vi "Board Info Report_v2.vi"(8 "error in (no error)":errorcluster, 11 "ControlBoard VISA":refnum<visa-resource-name>="ControlBoard") -> (0 "error out":errorcluster, 3 "Report":string)   [LabVIEW 2022 SP3]
uses:
  SupportVIs/VISA Flush IO Buffer Mask.ctl
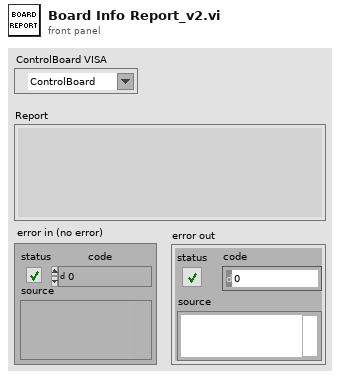
[diagram p1: front panel]
types:
  T1 = typedef "VISA Flush IO Buffer Mask.ctl" = u16
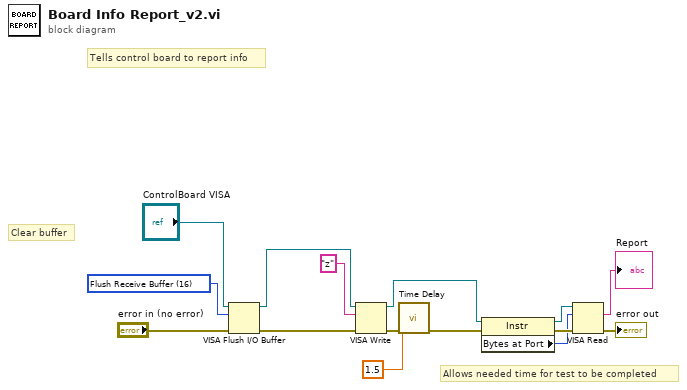
[diagram p0: block diagram]
diagram:
  w14 = T1 16 items=["Flush Receive Buffer"=16, "Write Transmit Buffer to Device"=32, "Flush Receive Buffer (No I/O)"=64, "Flush Transmit Buffer"=128] ("Mask")
  # "Allows needed time for test to be completed"
  # "Tells control board to report info"
  # "Clear buffer"
  n1 = VISA Flush I/O Buffer(VISA resource name="ControlBoard VISA", mask (16)=w14, error in (no error)="error in (no error)") -> (VISA resource name out=w12:refnum<visa-resource-name>, error out=w9:errorcluster)
  n2 = VISA Write(VISA resource name=w12, write buffer="z", error in (no error)=w9) -> (VISA resource name out=w7:refnum<visa-resource-name>, error out=w13:errorcluster)  [unwired: 1 out]
  n3 = call "Time Delay"("error in (no error)"=w13, "Delay Time (s)"=1.5) -> ("error out"=w8:errorcluster)  [unwired: 9 in]
  n4 = property class="Instr"(reference=w7, error in=w8) -> (reference out=w6:refnum<visa-resource-name>, error out=w5:errorcluster, "Bytes at Port"=w4:u32)
  n5 = VISA Read(VISA resource name=w6, byte count=w4, error in (no error)=w5) -> (read buffer=→"Report":string, error out=→"error out":errorcluster)  [unwired: 2 out]
